vi "File Error Handler.vi"(0 "FILE SYSTEM\nERROR CODE":i16) -> (1 "ERROR INDICATOR\nLED":bool, 2 "ERROR MESSAGE":string="No Error")   [LabVIEW 2021]
doc: "This VI takes an error number an outputs the appropriate error message for file I/O operations.\nScott Hannahs, FBNML, Jan 1992"
panel:
  in  "?":string="File directory full.\rDisk full.\rNo such volume.\rI/O error (bummers).\rBad file name or volume name (perhaps zero length).\rFile not open.\rLogical end-of-file reached during read operation\rAttempt to position before start of file\rMemory full (open) or file won't fit (load).\rToo many files open.  Only 12 files can be open simultaneously\rFile not found\rVolume is locked by a hardware setting.\rFile is locked.\rVolume is locked by a software setting.\rFile is busy; one or more files are open.\rFile already open.\rError in parameter list.  Parameters do not specify an existing volume, and there is no default volume (file manager), bad positioning informations (disk driver), or bad drive number (disk initialization package).\rPath reference number specifies nonexisiten access path."
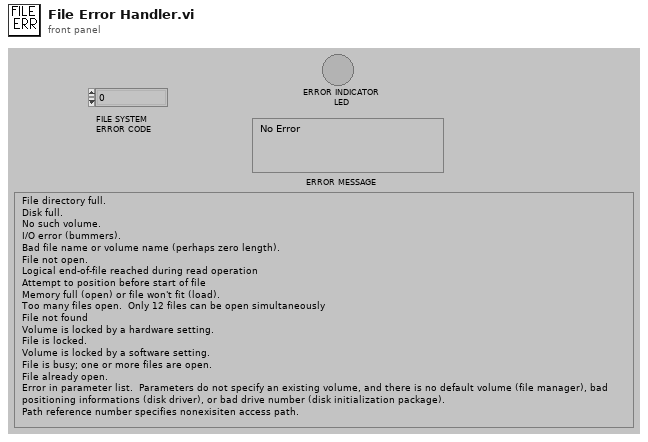
[diagram p1: front panel]
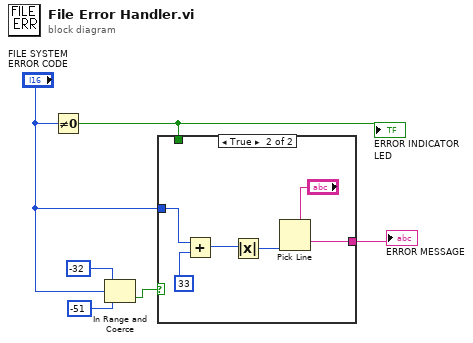
[diagram p0: block diagram]
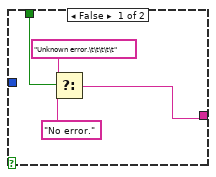
[diagram p2: hidden frame]
diagram:
  n1 = Not Equal To 0?(x="FILE SYSTEM\nERROR CODE") -> (x != 0?=w5:bool)
  "ERROR INDICATOR\nLED" <- w5
  n2 = In Range and Coerce(upper limit=-32, x="FILE SYSTEM\nERROR CODE", lower limit=-51) -> (In Range?=w4:bool)  [unwired: 1 out]
  n3 = case shown="True" w4 {
    tunnel: "FILE SYSTEM\nERROR CODE" -> [_ w12]
    tunnel: [w8 w15] -> w6
    tunnel: w5 -> [w7 _]
    frame False {
      n4 = Select(t="Unknown error.\t\t\t\t\t", s=w7, f="No error.") -> (s? t:f=w8:string)
    }
    frame True {
      n5 = Add(x=w12, y=i16 33) -> (x+y=w13:i16)
      n6 = Absolute Value(x=w13) -> (abs(x)=w14:i16)
      n7 = Pick Line(multi-line string="?", line index=w14) -> (output string=w15:string)  [unwired: 1 in]
    }
  }
  "ERROR MESSAGE" <- w6
